vi "CoordinateConvert_ArmToCartesian.vi"(3 "Wrist Angle (rad)":dbl, 4 "Radius (in)":dbl, 5 "Shoulder Angle (rad)":dbl) -> (0 "Wrist (rad)":dbl, 1 "Y (in)":dbl, 2 "X (in)":dbl)   [LabVIEW 2018]
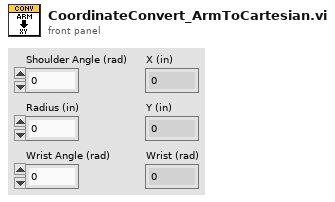
[diagram p1: front panel]
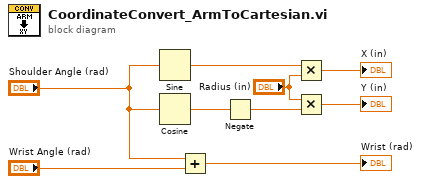
[diagram p0: block diagram]
diagram:
  n1 = Sine(x="Shoulder Angle (rad)") -> (sin(x)=w9:dbl)
  n2 = Cosine(x="Shoulder Angle (rad)") -> (cos(x)=w6:dbl)
  n3 = Add(x="Shoulder Angle (rad)", y="Wrist Angle (rad)") -> (x+y=→"Wrist (rad)":dbl)
  n4 = Negate(x=w6) -> (-x=w5:dbl)
  n5 = Multiply(x=w9, y="Radius (in)") -> (x*y=→"X (in)":dbl)
  n6 = Multiply(x="Radius (in)", y=w5) -> (x*y=→"Y (in)":dbl)
